vi "AutoDriveBack.vi"(8 "error in (no error)":errorcluster, 11 "RobotDriveDevRef":T1={"DevStatus"={"status"=FALSE, "code"=0, "source"=""}, "Motors[]"=[], "Square Inputs"=FALSE, "Max Output"=1.0, "Isochronous"=FALSE}) -> (0 "error out":errorcluster)   [LabVIEW 2013]
uses:
  <vilib>/Rock Robotics/WPI/RobotDrive/WPI_RobotDriveDevRef.ctl
  <vilib>/Rock Robotics/WPI/MotorControl/WPI_MotorControlDeviceRef.ctl
  <vilib>/Rock Robotics/SystemInterfaces/Typedef/FPGA_TypedefDigitalModule.ctl
  <vilib>/Rock Robotics/SystemInterfaces/DIO/FPGA_DIOPWMChannel.ctl
  <vilib>/Rock Robotics/WPI/PWM/WPI_PWMDeadband.ctl
  <vilib>/Rock Robotics/WPI/CAN/Jaguar/SubVIs/WPI_CANJaguar_ControlMode.ctl
  <vilib>/Rock Robotics/WPI/PWM/WPI_PWMTransform_ConPane.ctl
  <vilib>/addons/control/pid/pid.llb/PID Control Input Filter (DBL).vi
  <vilib>/addons/control/pid/pid.llb/PID (DBL).vi
  <vilib>/addons/control/pid/NI_PID_pid.lvlib
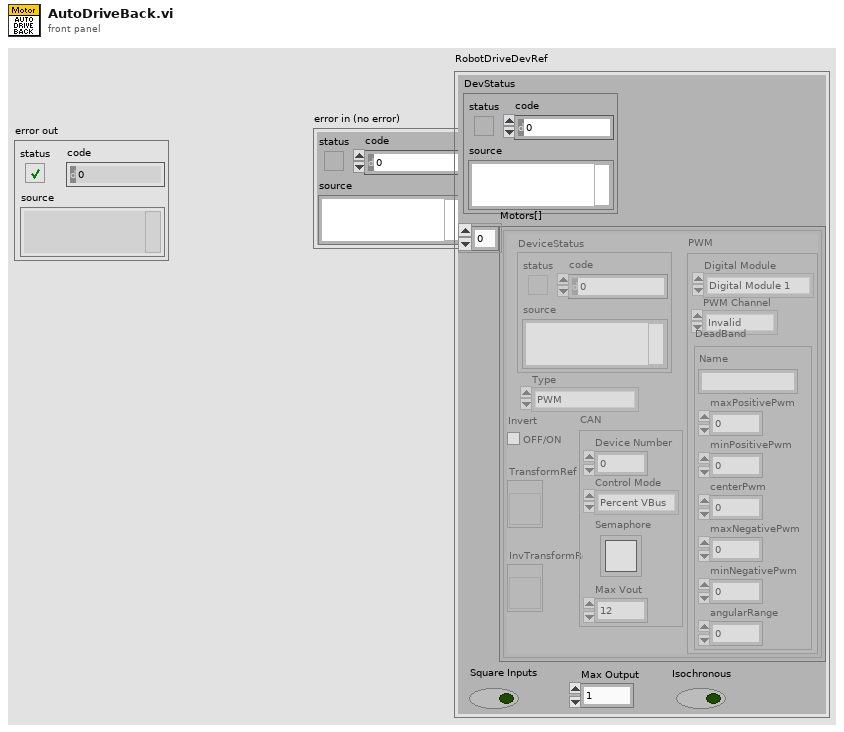
[diagram p1: front panel]
types:
  T1 = typedef "WPI_RobotDriveDevRef.ctl" = cluster{"DevStatus":errorcluster, "Motors[]":T2[], "Square Inputs":bool, "Max Output":dbl, "Isochronous":bool}
  T2 = typedef "WPI_MotorControlDeviceRef.ctl" = cluster{"DeviceStatus":errorcluster, "Type":enum16{"PWM", "CAN"}, "PWM":cluster{"Digital Module":T3, "PWM Channel":T4, "DeadBand":T5}, "CAN":cluster{"Device Number":u8, "Control Mode":T6, "Semaphore":T7, "Max Vout":dbl}, "Invert":bool, "TransformRef":T8, "InvTransformRef":T8}
  T3 = typedef "FPGA_TypedefDigitalModule.ctl" = enum16{"Digital Module 1", "Digital Module 2"}
  T4 = typedef "FPGA_DIOPWMChannel.ctl" = enum8{"PWM 1", "PWM 2", "PWM 3", "PWM 4", "PWM 5", "PWM 6", "PWM 7", "PWM 8", "PWM 9", "PWM 10", "Invalid"}
  T5 = typedef "WPI_PWMDeadband.ctl" = cluster{"Name":string, "maxPositivePwm":i32, "minPositivePwm":i32, "centerPwm":i32, "maxNegativePwm":i32, "minNegativePwm":i32, "angularRange":u16}
  T6 = typedef "WPI_CANJaguar_ControlMode.ctl" = enum8{"Percent VBus", "Current", "Speed", "Position", "Voltage"}
  T7 = typedef "Semaphore RefNum" = refnum<k1>
  T8 = typedef "WPI_PWMTransform_ConPane.ctl" = refnum<vi>
  T9 = cluster{"proportional gain (Kc)":dbl, "integral time (Ti, min)":dbl, "derivative time (Td, min)":dbl}
  T10 = typedef "WPI_EncoderDevRef.ctl" = cluster{"DevStatus":errorcluster, "EncoderIndex":T11, "CounterIndex":T12, "DistancePerCount":dbl, "Decoding Type":T13}
  T11 = typedef "FPGA_EncoderIdx.ctl" = enum8{"Enc 0", "Enc 1", "Enc 2", "Enc 3", "Invalid"}
  T12 = typedef "FPGA_CounterCtrSystemIndex.ctl" = enum8{"Ctr 0", "Ctr 1", "Ctr 2", "Ctr 3", "Ctr 4", "Ctr 5", "Ctr 6", "Ctr 7", "Invalid"}
  T13 = typedef "WPI_EncoderType.ctl" = enum16{"1x", "2x", "4x"}
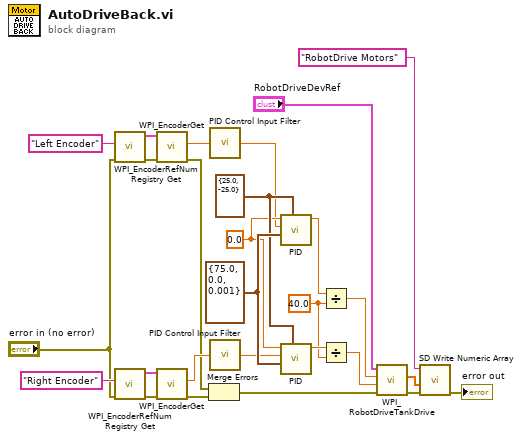
[diagram p0: block diagram]
diagram:
  w5 = 0.0 ("setpoint")
  w6 = cluster{"output high":dbl, "output low":dbl} {"output high"=25.0, "output low"=-25.0} ("output range")
  w7 = 40.0 ("y")
  w27 = T9 {"proportional gain (Kc)"=75.0, "integral time (Ti, min)"=0.0, "derivative time (Td, min)"=0.001} ("PID gains")
  n1 = call <vilib>:"WPI_EncoderRefNum Registry Get.vi"("error in (no error)"="error in (no error)", "refnum name"="Left Encoder") -> ("error out"=w21:errorcluster, "EncoderDevRef"=w22:T10)  [unwired: 8 in]
  n2 = call <vilib>:"WPI_EncoderRefNum Registry Get.vi"("error in (no error)"="error in (no error)", "refnum name"="Right Encoder") -> ("error out"=w23:errorcluster, "EncoderDevRef"=w24:T10)  [unwired: 8 in]
  n3 = call <vilib>:"WPI_EncoderGet.vi"("error in (no error)"=w21, "EncoderDevRef"=w22) -> ("error out"=w16:errorcluster, "Distance"=w19:dbl)  [unwired: 4 in, 4 out]
  n4 = call <vilib>:"WPI_EncoderGet.vi"("error in (no error)"=w23, "EncoderDevRef"=w24) -> ("error out"=w17:errorcluster, "Distance"=w18:dbl)  [unwired: 4 in, 4 out]
  n5 = Merge Errors(w16, w17) -> (w15:errorcluster)
  n6 = call-poly <vilib>:"PID Control Input Filter.vi"("input"=w19) -> ("output"=w2:dbl)  [unwired: 4 in]
  n7 = call-poly <vilib>:"PID Control Input Filter.vi"("input"=w18) -> ("output"=w1:dbl)  [unwired: 4 in]
  n8 = call-poly <vilib>:"PID.vi"("output range"=w6, "PID gains"=w27, "process variable"=w2, "setpoint"=w5) -> ("output"=w8:dbl)  [unwired: 6 in, 1 out]
  n9 = call-poly <vilib>:"PID.vi"("output range"=w6, "PID gains"=w27, "process variable"=w1, "setpoint"=w5) -> ("output"=w9:dbl)  [unwired: 6 in, 1 out]
  n10 = Divide(x=w8, y=w7) -> (x/y=w10:dbl)
  n11 = Divide(x=w9, y=w7) -> (x/y=w11:dbl)
  n12 = call <vilib>:"WPI_RobotDriveTankDrive.vi"("error in (no error)"=w15, "Right axis value"=w11, "Left axis value"=w10, "RobotDriveDevRef"="RobotDriveDevRef") -> ("error out"=w14:errorcluster, "Motor Values"=w13:dbl[])  [unwired: 5 in, 1 out]
  n13 = call <vilib>:"SD Write Numeric Array.vi"("error in"=w14, "Numeric Array"=w13, "Name"="RobotDrive Motors") -> ("error out"=→"error out":errorcluster)  [unwired: 7 in, 1 out]
